vi "PM100D_Initialize.vi"() -> (0 "error out":errorcluster, 1 "Instrument":string, 2 "VISA out":refnum<visa-resource-name>, 4 "SN":string)   [LabVIEW 2013]
doc: "This VI scans for connected devices, that can be selected in a dialog box. Next steps\n- setting timeout\n- performing identification query\n- configuring the operation register to '512'; flag gets to HI when a new measurement value is ready to fetch\n- clear operation register"
uses:
  <vilib>/Instr/_visa.llb/VISA Find Search Mode.ctl
  <vilib>/Instr/_visa.llb/VISA Configure Serial Port (Instr).vi
panel:
  out "List of Visa devices":string[](array[string])
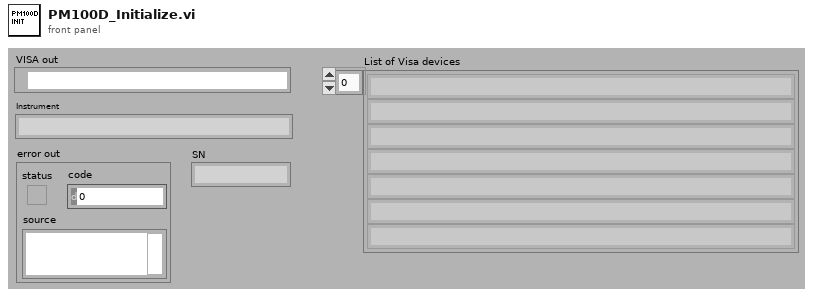
[diagram p1: front panel]
types:
  T1 = typedef "VISA Find Search Mode.ctl" = u32
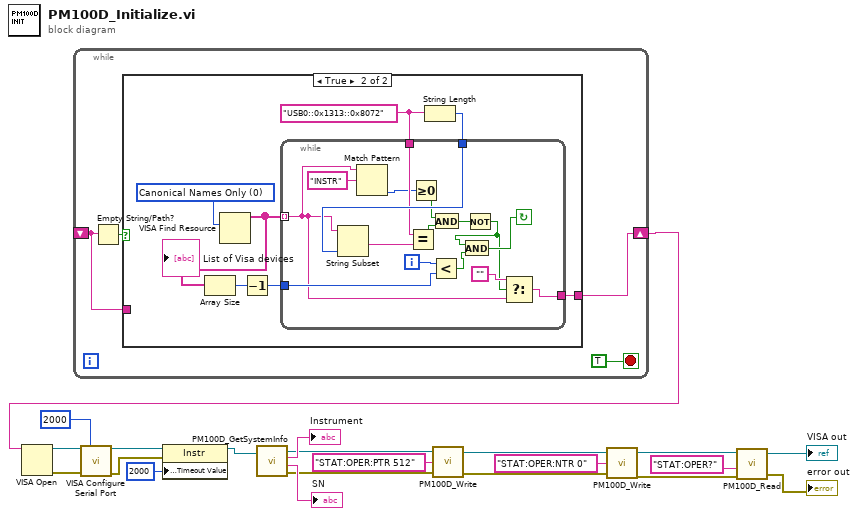
[diagram p0: block diagram]
diagram:
  n1 = while {
    shift-right: [w25] -> w6
    shift-left: _ -> [w23]
    stop <- TRUE stop-if-true
    n2 = Empty String/Path?(string/path=w23) -> (empty?=w24:bool)
    n3 = case shown="True" w24 {
      tunnel: [w26 w27] -> w25
      tunnel: w23 -> [w26 _]
      frame False {
      }
      frame True {
        w33 = T1 0 items=["Canonical Names Only"=0, "Aliases Only"=1, "Include Matching Aliases"=2, "Include All Aliases"=4] ("Search Mode")
        w31 = "USB0::0x1313::0x8072" ("element")
        n4 = VISA Find Resource(10:w33) -> (3:w30:string[])  [unwired: 1 in, 3 out]
        "List of Visa devices" <- w30
        n5 = Array Size(array=w30) -> (size(s)=w29:i32)
        n6 = Decrement(x=w29) -> (x-1=w28:i32)
        n7 = String Length(string=w31) -> (length=w32:i32)
        n8 = while {
          tunnel: w32 -> [w49]
          tunnel: w30 -> [w39] mode=indexing
          tunnel: w31 -> [w48]
          tunnel: w28 -> [w45]
          tunnel: [w42] -> w27
          i -> [w46]
          stop <- w43 continue-if-true
          n9 = String Subset(string=w39, length (rest)=w49) -> (substring=w47:string)  [unwired: 1 in]
          n10 = Match Pattern(string=w39, regular expression="INSTR") -> (offset past match=w38:i32)  [unwired: 1 in, 3 out]
          n11 = Equal?(x=w48, y=w47) -> (x = y?=w36:bool)
          n12 = Greater Or Equal To 0?(x=w38) -> (x >= 0?=w37:bool)
          n13 = Less?(x=w46, y=w45) -> (x < y?=w44:bool)
          n14 = And(x=w37, y=w36) -> (x .and. y?=w35:bool)
          n15 = Not(x=w35) -> (.not. x?=w34:bool)
          n16 = And(x=w34, y=w44) -> (x .and. y?=w43:bool)
          n17 = Select(t="", s=w34, f=w39) -> (s? t:f=w42:string)
        }
      }
    }
  }
  n18 = VISA Open(VISA resource name=w6) -> (VISA resource name=w5:refnum<visa-resource-name>, error out=w4:errorcluster)  [unwired: 1 in, 3 out]
  n19 = call-poly "VISA Configure Serial Port"("VISA resource name"=w5, "timeout (10sec)"=u32 2000, "error in (no error)"=w4) -> ("VISA resource name out"=w3:refnum<visa-resource-name>, "error out"=w2:errorcluster)  [unwired: 11 in]
  n20 = property class="Instr"(reference=w3, error in=w2, "General Settings:Timeout Value"=u32 2000) -> (reference out=w18:refnum<visa-resource-name>)  [unwired: 1 out]
  n21 = call "PM100D_GetSystemInfo.vi"("VISA in"=w18) -> ("VISA out"=w16:refnum<visa-resource-name>, "Instrument"=→"Instrument":string, "SN"=→"SN":string, "error out"=w14:errorcluster)  [unwired: 1 in]
  n22 = call "PM100D_Write.vi"("error in (no error)"=w14, "Command"="STAT:OPER:PTR 512", "VISA in"=w16) -> ("error out"=w13:errorcluster, "VISA out"=w15:refnum<visa-resource-name>)
  n23 = call "PM100D_Write.vi"("error in (no error)"=w13, "Command"="STAT:OPER:NTR 0", "VISA in"=w15) -> ("error out"=w7:errorcluster, "VISA out"=w11:refnum<visa-resource-name>)
  n24 = call "PM100D_Read.vi"("error in (no error)"=w7, "Command"="STAT:OPER?", "VISA in"=w11) -> ("error out"=→"error out":errorcluster, "VISA out"=→"VISA out":refnum<visa-resource-name>)  [unwired: 2 out]
